vi "doTimeSeries.vi"(0 "period_s":dbl=3600.0, 1 "pixel_dwell_ms":dbl=1.0 caption="Dwell time ms:", 2 "autofocus":bool, 5 "date_stop":timestamp=timestamp(3557127149.3091764 s since 1904-01-01), 7 "pos_start_xy":cluster{"pos_start_x":dbl, "pos_start_y":dbl}, 9 "image_size_x_um":dbl=150.0, 11 "frame_size_x_px":i32=100, 12 "pos_start":enum32{"bottom-left", "center"}(ring), 13 "scan_direction":enum32{"0", "1"}(radio)=enum."1" caption="Scan direction:", 14 "IntensityGraph in":refnum<vi>) -> ()   [LabVIEW 2014]
panel:
  out "time_remaining":string
  out "image_number":i32
  in  "focus-pixel_dwell_ms":dbl=0.3 caption="focus Dwell time ms:"
  in  "focus-frame_size_x_px":i32=50 caption="frame_size_x_px"
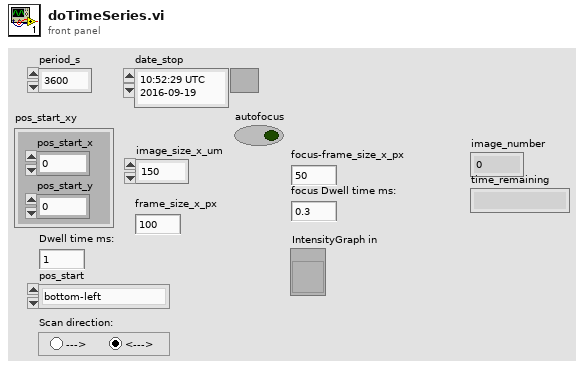
[diagram p1: front panel]
types:
  T1 = cluster{"image_size_x_um":dbl, "image_size_x_um":dbl}
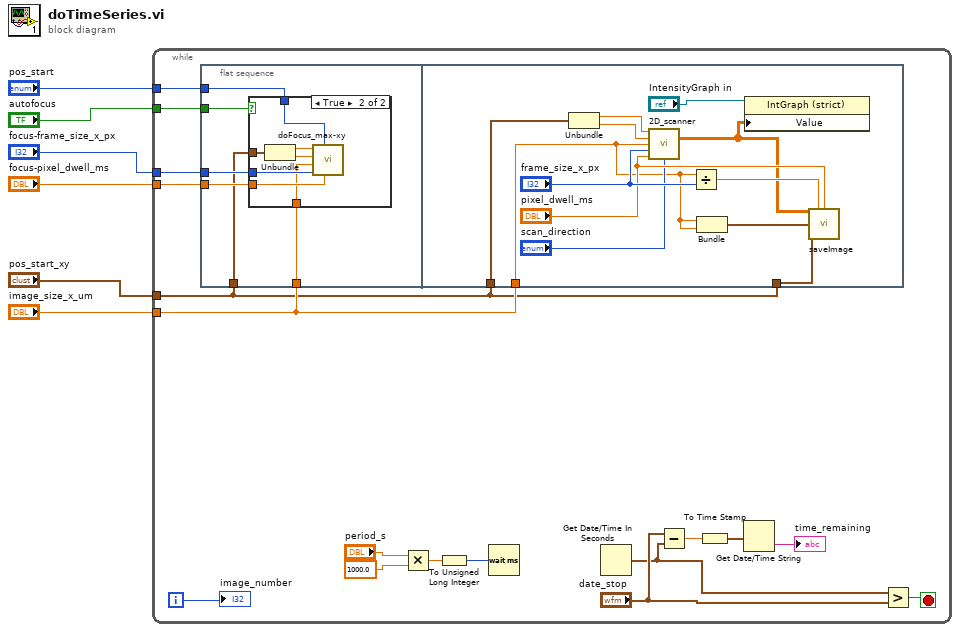
[diagram p0: block diagram]
diagram:
  n1 = while {
    tunnel: "pos_start" -> [w12]
    tunnel: "image_size_x_um" -> [w9]
    tunnel: "autofocus" -> [w13]
    tunnel: "pos_start_xy" -> [w8]
    tunnel: "focus-pixel_dwell_ms" -> [w11]
    tunnel: "focus-frame_size_x_px" -> [w10]
    i -> [w18]
    stop <- w23 stop-if-true
    n2 = flat-sequence {
      tunnel: w13 -> [w29]
      tunnel: w12 -> [w28]
      tunnel: w11 -> [w27]
      tunnel: w10 -> [w26]
      tunnel: w9 -> [w25]
      tunnel: w8 -> [w24]
      tunnel: w8 -> [w45]
      tunnel: w9 -> [w42]
      tunnel: w8 -> [w39]
      frame #0 {
        n3 = case shown="True" w29 {
          tunnel: w28 -> [_ w36]
          tunnel: w27 -> [_ w35]
          tunnel: w26 -> [_ w34]
          tunnel: w25 -> [_ w33]
          tunnel: w24 -> [_ w30]
          frame False {
          }
          frame True {
            n4 = Unbundle(w30) -> ("pos_start_x"=w32:dbl, "pos_start_y"=w31:dbl)
            n5 = call "doFocus_max-xy.vi"("pixel_dwell_ms"=w35, "pos_start"=w36, "frame_size_x_px"=w34, "image_size_x_um"=w33, "pos-start_y"=w31, "pos-start_x"=w32) -> ()  [unwired: 4 in, 2 out]
          }
        }
      }
      frame #1 {
        n6 = Unbundle(w39) -> ("pos_start_x"=w40:dbl, "pos_start_y"=w41:dbl)
        n7 = call "2D_scanner.vi"("pos-start_x"=w40, "pos-start_y"=w41, "image_size_x_um"=w42, "frame_size_x_px"="frame_size_x_px", "pixel_dwell_ms"="pixel_dwell_ms", "scan_direction"="scan_direction") -> ("image_out"=w38:dbl[][])  [unwired: 9 in]
        n8 = Divide(x=w42, y="frame_size_x_px") -> (x/y=w44:dbl)
        n9 = Bundle("image_size_x_um"=w42, "image_size_x_um"=w42) -> (w43:T1)  [unwired: 1 in]
        n10 = property class="IntGraph (strict)"(reference="IntensityGraph in", "Value"=w38) -> ()  [unwired: 1 in, 2 out]
        n11 = call "saveImage.vi"("image"=w38, "image-step_size"=w44, "image-dwell_time"="pixel_dwell_ms", "image_start_xyz"=w45, "image_size_xy"=w43) -> ()  [unwired: 10 in, 1 out]
      }
    }
    n12 = Multiply(x="period_s", y=1000.0) -> (x*y=w20:dbl)
    n13 = To Unsigned Long Integer(number=w20) -> (unsigned 32bit integer=w21:u32)
    n14 = Wait (ms)(milliseconds to wait=w21) -> ()  [unwired: 1 out]
    n15 = Get Date/Time In Seconds() -> (seconds since 1Jan1904=w16:timestamp)
    n16 = Subtract(x="date_stop", y=w16) -> (x-y=w15:dbl)
    n17 = To Time Stamp(1:w15) -> (0:w14:timestamp)
    n18 = Get Date/Time String(seconds (now)=w14) -> (time string=→"time_remaining":string)  [unwired: 2 in, 1 out]
    n19 = Greater?(x=w16, y="date_stop") -> (0:w23:bool)
    "image_number" <- w18
  }
